vi "AcknowledgeAll.vi"(8 "error in (no error)":errorcluster, 11 "controller in":refnum<k24>) -> (0 "error out":errorcluster, 3 "controller out":refnum<k24>)   [LabVIEW 2019]
uses:
  C:/Users/patrick/Documents/GitHub/Aerotech-Delay-Line/lvsrc/Aerotech-Ensemble-LabVIEW/2010-5.6/Bin/Aerotech.Ensemble.dll
  Bin/Aerotech.Ensemble.dll
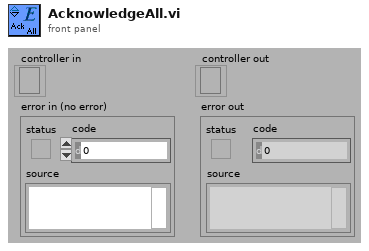
[diagram p1: front panel]
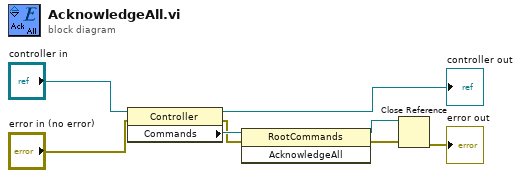
[diagram p0: block diagram]
diagram:
  n1 = property class="Controller"(reference="controller in", error in="error in (no error)") -> (reference out=→"controller out":refnum<k24>, error out=w4:errorcluster, "Commands"=w5:refnum<k24>)
  n2 = invoke class="RootCommands" method="AcknowledgeAll"(reference=w5, error in=w4) -> (reference out=w2:refnum<k24>, error out=w1:errorcluster)  [unwired: 1 in, 1 out]
  n3 = Close Reference(reference=w2, error in (no error)=w1) -> (error out=→"error out":errorcluster)
